vi "GetSwerveAbsoluteAzimuth.vi"(0 "Relative Position (Raw Sensor Units)":i32) -> (1 "Azimuth Position (deg) [-180,+180]":dbl, 2 "Current Unwrapped Angle (deg) [-Inf,+Inf]":dbl)   [LabVIEW 2020]
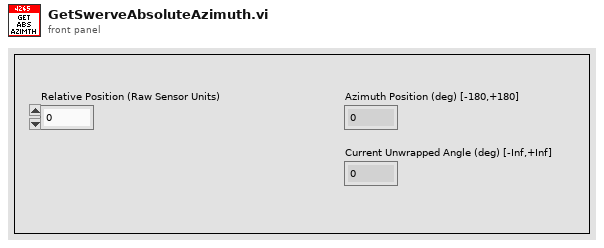
[diagram p1: front panel]
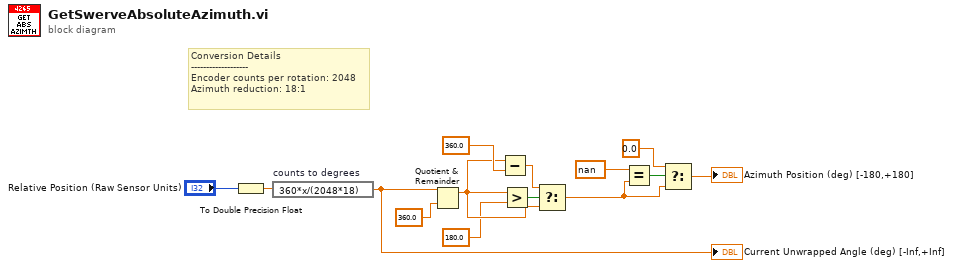
[diagram p0: block diagram]
diagram:
  # "Conversion Details\n-------------------\nEncoder counts per rotation: 2048\nAzimuth reduction: 18:1"
  n1 = To Double Precision Float(number="Relative Position (Raw Sensor Units)") -> (double precision float=w13:dbl)
  n2 = expression code="360*x/(2048*18)" "counts to degrees"(w13) -> (w1:dbl)
  "Current Unwrapped Angle (deg) [-Inf,+Inf]" <- w1
  n3 = Quotient & Remainder(x=w1, y=360.0) -> (x-y*floor(x/y)=w10:dbl)  [unwired: 1 out]
  n4 = Subtract(x=w10, y=360.0) -> (x-y=w11:dbl)
  n5 = Greater?(x=w10, y=180.0) -> (0:w9:bool)
  n6 = Select(t=w11, s=w9, f=w10) -> (s? t:f=w4:dbl)
  n7 = Equal?(x=nan, y=w4) -> (x = y?=w5:bool)
  n8 = Select(t=0.0, s=w5, f=w4) -> (s? t:f=→"Azimuth Position (deg) [-180,+180]":dbl)
